vi "Update_DA.vi"(8 "error in (no error)":errorcluster, 10 "RAW":bool, 11 "Sig_DA in":refnum<class "Sig_DA.lvclass">) -> (0 "error out":errorcluster, 2 "CURR":bool, 3 "Sig_DA out":refnum<class "Sig_DA.lvclass">)   [LabVIEW 2019, in "Sig_DA.lvclass"]
uses:
  Sig_DA.lvclass
  D:/H4000/src/Proccess_class/Proccess.lvclass
  Sig_DA.lvclass/Sig_DA.ctl
  Proccess_class/Proccess.lvclass/Proccess.ctl
  Proccess_class/Read TagName.vi
  Proccess_class/Read Logger.vi
  Logger_class/WriteEvent.vi
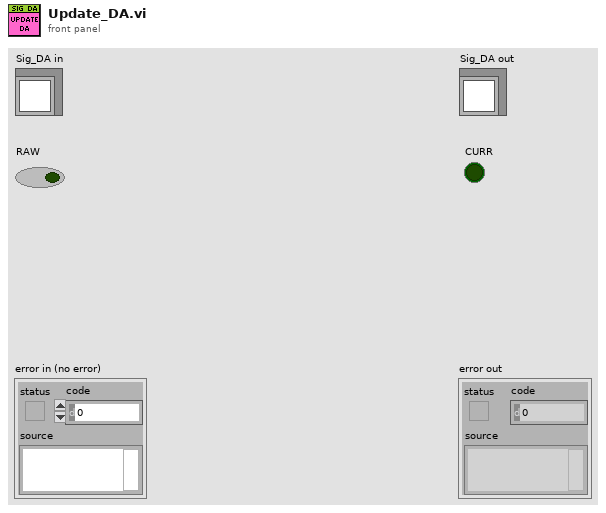
[diagram p1: front panel]
types:
  T1 = typedef "bool_data.ctl" = cluster{"CURR":bool, "RAW_PREV":bool, "millisecond timer value":u32}
  T2 = typedef "bool_setting.ctl" = cluster{"TON_ms":u32, "TOFF_ms":u32}
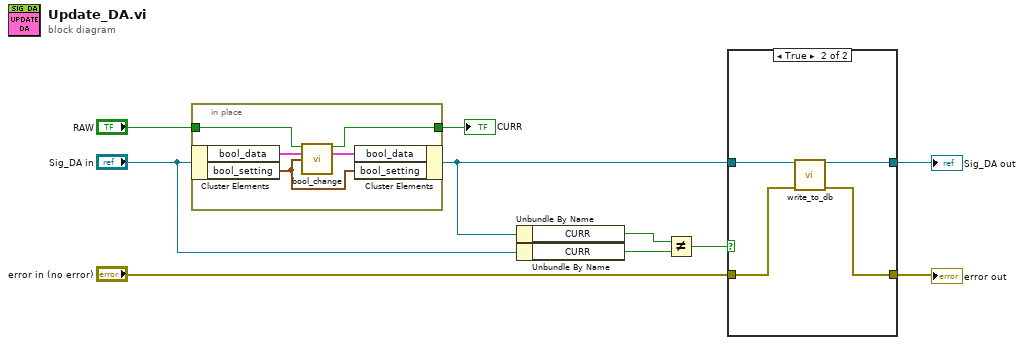
[diagram p0: block diagram]
diagram:
  n1 = in-place {
    in-place-border: "RAW" -> [w12]
    in-place-border: [w11] -> w9
    n2 = in-place-cluster #1("Sig_DA in") -> ("bool_data"=w15:T1, "bool_setting"=w13:T2)
    n3 = call "bool_change.vi"("RAW"=w12, "bool_data_in"=w15, "bool_setting"=w13) -> ("CURR"=w11:bool, "bool_data_out"=w14:T1)  [unwired: 11 in]
    n4 = in-place-cluster #1("bool_data"=w14, "bool_setting"=w13) -> (w4:refnum<class "Sig_DA.lvclass">)
  }
  "CURR" <- w9
  n5 = Unbundle By Name(w4) -> ("CURR"=w6:bool)
  n6 = Unbundle By Name("Sig_DA in") -> ("CURR"=w7:bool)
  n7 = Not Equal?(x=w6, y=w7) -> (x != y?=w5:bool)
  n8 = case shown="True" w5 {
    tunnel: w4 -> [w17 w21]
    tunnel: [w17 w20] -> w3
    tunnel: "error in (no error)" -> [w16 w19]
    tunnel: [w16 w18] -> w1
    frame False {
    }
    frame True {
      n9 = call "write_to_db.vi"("reference in"=w21, "error in (no error)"=w19) -> ("reference out"=w20:refnum<class "Sig_DA.lvclass">, "error out"=w18:errorcluster)  [unwired: 12 in]
    }
  }
  "error out" <- w1
  "Sig_DA out" <- w3
